vi "Array Test.vi"() -> ()   [LabVIEW 2017]
panel:
  out "Output String":string
  out "array":dbl[](array[numeric])
  out "appended array":dbl[][](array[numeric])
  out "Iteration":i32
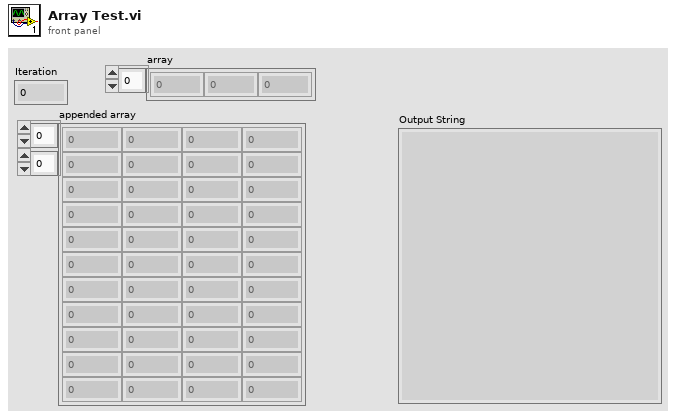
[diagram p1: front panel]
types:
  T1 = cluster{dbl, "number: 0 to 1":dbl, "number: 0 to 1":dbl}
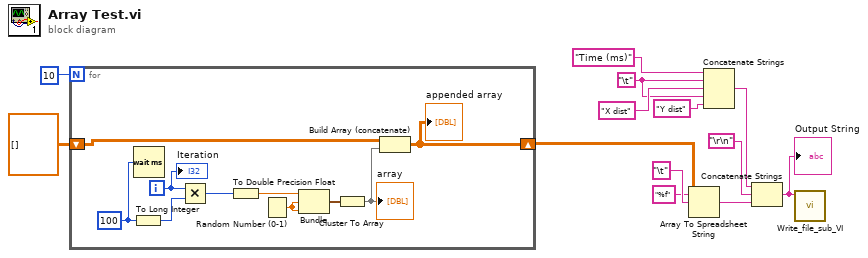
[diagram p0: block diagram]
diagram:
  w8 = "\t"
  n1 = for {
    N: 10 -> [_]
    shift-right: [w14] -> w11
    shift-left: dbl[][] [] -> [w16]
    i -> [w23]
    w22 = u32 100
    n2 = To Long Integer(number=w22) -> (32bit integer=w21:i32)
    n3 = Wait (ms)(milliseconds to wait=w22) -> ()  [unwired: 1 out]
    n4 = Multiply(x=w23, y=w21) -> (x*y=w19:i32)
    n5 = To Double Precision Float(number=w19) -> (double precision float=w17:dbl)
    n6 = Random Number (0-1)() -> (number: 0 to 1=w18:dbl)
    n7 = Bundle(w17, "number: 0 to 1"=w18, "number: 0 to 1"=w18) -> (w20:T1)  [unwired: 1 in]
    n8 = Cluster To Array(cluster=w20) -> (array=w15:dbl[])
    "array" <- w15
    n9 = Build Array (concatenate)(w16, w15) -> (w14:dbl[][])
    "appended array" <- w14
    "Iteration" <- w23
  }
  n10 = Array To Spreadsheet String(delimiter (Tab)="\t", array=w11, 3:"%f" ("format string")) -> (spreadsheet string=w4:string)
  n11 = Concatenate Strings("Time (ms)", w8, "X dist", w8, "Y dist") -> (w6:string)
  n12 = Concatenate Strings(w6, "\r\n", w4) -> (w1:string)
  "Output String" <- w1
  n13 = call "Write_file_sub_VI.vi"("Output String"=w1) -> ()  [unwired: 9 in, 2 out]
